vi "getPromedio.vi"(2 "N":i32, 3 "Contraste":dbl, 4 "Reset":bool) -> (0 "Llego a N?":bool, 1 "Contraste Promedio":dbl)   [LabVIEW 2010]
uses:
  <vilib>/Analysis/NI_AALBase.lvlib
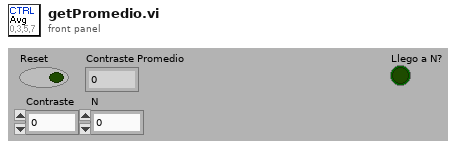
[diagram p1: front panel]
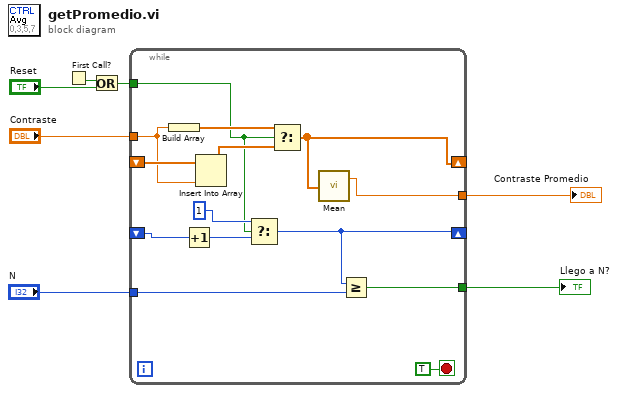
[diagram p0: block diagram]
diagram:
  n1 = First Call?() -> (First Call?: T/F=w7:bool)
  n2 = Or(x=w7, y="Reset") -> (x .or. y?=w5:bool)
  n3 = while {
    tunnel: w5 -> [w13]
    shift-right: [w20] -> _
    shift-left: _ -> [w17]
    tunnel: "Contraste" -> [w16]
    tunnel: [w19] -> w3
    shift-right: [w10] -> _
    shift-left: _ -> [w12]
    tunnel: "N" -> [w9]
    tunnel: [w8] -> w1
    stop <- TRUE stop-if-true
    n4 = Build Array(w16) -> (w18:dbl[])
    n5 = Increment(x=w12) -> (x+1=w11:i32)
    n6 = Insert Into Array(array=w17, new element=w16) -> (w15:dbl[])  [unwired: 1 in]
    n7 = Select(t=1, s=w13, f=w11) -> (s? t:f=w10:i32)
    n8 = Select(t=w18, s=w13, f=w15) -> (s? t:f=w20:dbl[])
    n9 = call <vilib>:"Mean.vi"("X"=w20) -> ("mean"=w19:dbl)  [unwired: 1 out]
    n10 = Greater Or Equal?(x=w10, y=w9) -> (x >= y?=w8:bool)
  }
  "Contraste Promedio" <- w3
  "Llego a N?" <- w1
